vi "SelectColor.vi"(3 "Image":T1 {"Dialogs" format="%.0b"}) -> (0 "Pen":u32(colorbox)=16777217 caption="Color", 1 "Image":T1 {"Dialogs" format="%.0b"})   [LabVIEW 2024]
doc: "This VI pops up a window where the user can select a region of interest."
uses:
  <userlib>/ImageProcessing/QTLIB_2595_LV86/QT_Image.ctl
  <vilib>/Utility/cursorutil.llb/Set Cursor (Icon Pict).vi
panel:
  in  "OK":bool
  out "Display":picture caption="new picture"
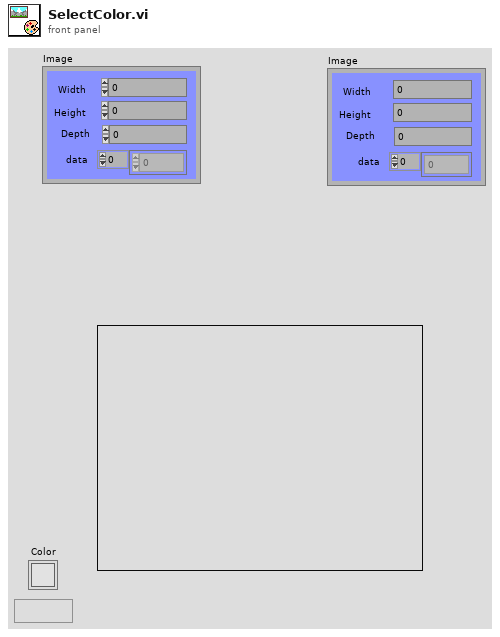
[diagram p1: front panel]
types:
  T1 = typedef "QT_Image.ctl" = cluster{"Width":i32, "Height":i32, "Depth":i32, "data":u8[], "Compressed data":u8[], "Color table":u32[], "Duration":i32, "Options":i32, "Timestamp":i32, "ID":i32, "Reserved":i32, "Dialogs":u32}
  T2 = typedef "LVRectTypeDef.ctl" = cluster{"left":i16, "top":i16, "right":i16, "bottom":i16}
  T3 = typedef "LVMouseTypeDef.ctl" = cluster{"Mouse Position":cluster{"X":i32, "Y":i32}, "Mouse Modifiers":cluster{"Button Down":bool, "Shift Mod":bool, "Menu Mod":bool, "Option Mod":bool}}
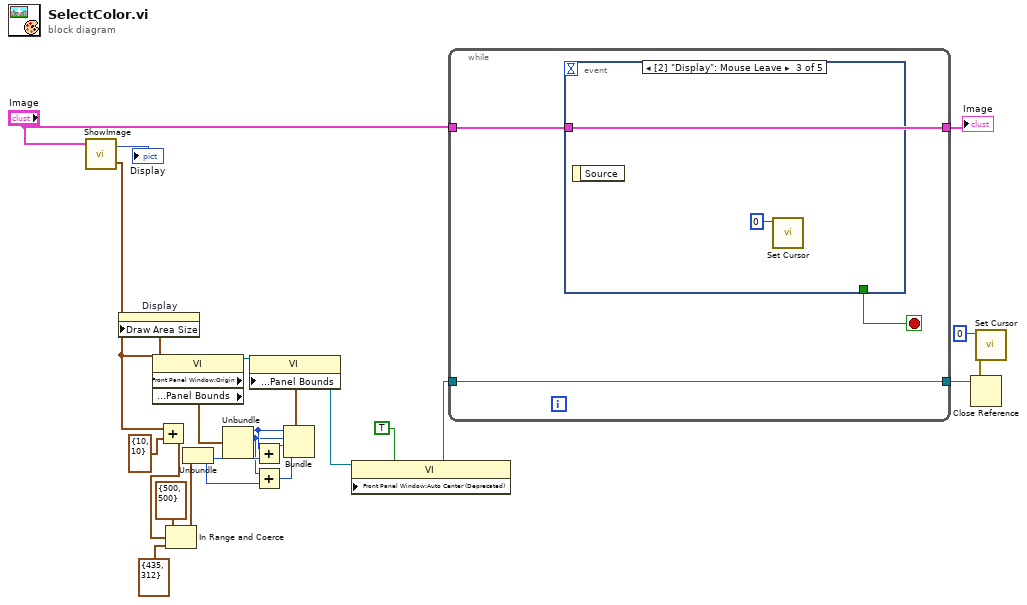
[diagram p0: block diagram]
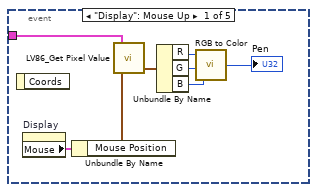
[diagram p2: hidden frame]
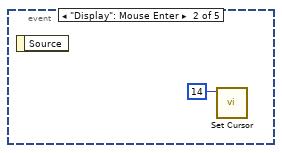
[diagram p3: hidden frame]
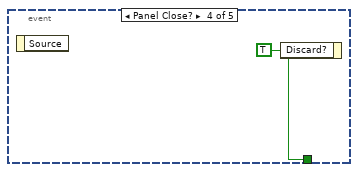
[diagram p4: hidden frame]
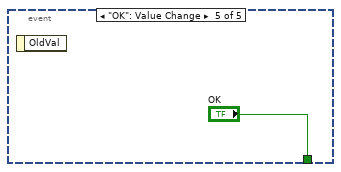
[diagram p5: hidden frame]
diagram:
  n1 = call <userlib>:"ShowImage.vi"("Image"="Image") -> ("dimensions"=w4:cluster{"Witdh":i32, "Height":i32}, "image"=→"Display":picture)  [unwired: 2 in]
  n2 = property on="Display" class="Pict"("Draw Area Size"=w4) -> ()  [unwired: 2 in, 2 out]
  n3 = property class="VI" props=["Front Panel Window:Origin", "Front Panel Window:Panel Bounds"]() -> (reference out=w22:refnum<vi>, "Front Panel Window:Panel Bounds"=w16:T2)  [unwired: 2 in, 2 out]
  n4 = Add(x=w4, y=cluster{i32, i32} {10, 10} ("x+y")) -> (x+y=w7:cluster{i32, i32})
  n5 = In Range and Coerce(upper limit=cluster{i32, i32} {500, 500}, x=w7, lower limit=cluster{i32, i32} {435, 312} ("x+y")) -> (coerced(x)=w6:cluster{i32, i32})  [unwired: 1 out]
  n6 = Unbundle(w6) -> (w13:i32, w12:i32)
  n7 = Unbundle(w16) -> ("left"=w11:i16, "top"=w10:i16)  [unwired: 2 out]
  n8 = Add(x=w11, y=w13) -> (x+y=w15:i32)
  n9 = Add(x=w10, y=w12) -> (x+y=w14:i32)
  n10 = Bundle("left"=w11, "top"=w10, w15, w14) -> (w20:cluster{"left":i16, "top":i16, i32, i32})  [unwired: 1 out]
  n11 = property class="VI"(reference=w22, "Front Panel Window:Panel Bounds"=w20) -> (reference out=w18:refnum<vi>)  [unwired: 1 in, 1 out]
  n12 = property class="VI"(reference=w18, "Front Panel Window:Auto Center (Deprecated)"=TRUE ("Front Panel Window:Auto Center")) -> (reference out=w19:refnum<vi>)  [unwired: 1 in, 1 out]
  n13 = while {
    tunnel: [w25] -> w23
    tunnel: w19 -> [w25]
    tunnel: [w27] -> w24
    tunnel: "Image" -> [w27]
    stop <- w26 stop-if-true
    n14 = event shown="[2] \"Display\": Mouse Leave" {
      selector: _ -> [_ _ _ _ _]
      dyn-events: _ -> [_ _ _ _ _]
      timeout: _ -> [_ _ _ _ _]
      tunnel: w27 -> [w35 _ _ _ _]
      tunnel: [_ _ _ w38 "OK"] -> w26
      event "Display": Mouse Up {
        n15 = event-data() -> ()  [unwired: 1 in, 1 out]
        n16 = property on="Display" class="Pict"() -> ("Mouse"=w29:T3)  [unwired: 2 in, 2 out]
        n17 = Unbundle By Name(w29) -> ("Mouse Position"=w28:cluster{"X":i32, "Y":i32})
        n18 = call <userlib>:"LV86_Get Pixel Value.vi"("Position"=w28, "Image In"=w35) -> ("RGB"=w34:cluster{"R":u32, "G":u32, "B":u32})  [unwired: 1 in, 2 out]
        n19 = Unbundle By Name(w34) -> ("R"=w33:u32, "G"=w32:u32, "B"=w31:u32)
        n20 = call <vilib>:"RGB to Color.vi"("B"=w31, "G"=w32, "R"=w33) -> ("Color"=→"Pen":u32)
      }
      event "Display": Mouse Enter {
        n21 = event-data() -> ()  [unwired: 1 in, 1 out]
        n22 = call-poly <vilib>:"Set Cursor.vi"("icon"=u16 14) -> ()  [unwired: 9 in, 2 out]
      }
      event "Display": Mouse Leave {
        n23 = event-data() -> ()  [unwired: 1 in, 1 out]
        n24 = call-poly <vilib>:"Set Cursor.vi"("icon"=u16 0) -> ()  [unwired: 9 in, 2 out]
      }
      event Panel Close? {
        w38 = TRUE ("Discard?")
        n25 = event-data() -> ()  [unwired: 1 in, 1 out]
        n26 = event-data("Discard?"=w38) -> ()  [unwired: 1 in, 1 out]
      }
      event "OK": Value Change {
        n27 = event-data() -> ()  [unwired: 1 in, 1 out]
      }
    }
  }
  "Image" <- w24
  n28 = Close Reference(reference=w23) -> (error out=w1:errorcluster)  [unwired: 1 in]
  n29 = call-poly <vilib>:"Set Cursor.vi"("error in (no error)"=w1, "icon"=u16 0) -> ()  [unwired: 8 in, 2 out]
